vi "I-V_Juliet.vi"() -> ()   [LabVIEW 2013]
uses:
  <vilib>/Utility/file.llb/Read From Spreadsheet File (DBL).vi
panel:
  in  "I-Min":dbl=0.006 format="%#_6e"
  out "dV/dI-I":cluster{dbl[], dbl[]}(graph) caption="XY Graph"
  out "I-V":cluster{dbl[], dbl[]}(graph) caption="XY Graph"
  in  "Measure I-V":bool
  in  "File name":string="C:\\User Data\\Guang\\20201217 Harry 42C\\IV"
  in  "Delta [A]":dbl=1e-05 format="%#_6e"
  in  "Step [A]":dbl=3e-05 format="%#_6e"
  in  "Abort Conductance":bool
  in  "Keithley":refnum<visa-resource-name>="GPIB0::20::INSTR"
  in  "Arm Conductance":bool
  in  "I-Max [A]":dbl=-0.006 format="%#_6e"
  in  "Delay [sec]":dbl=0.002 format="%#_6e"
  in  "Compliance [V]":dbl=10.0 format="%#_6f"
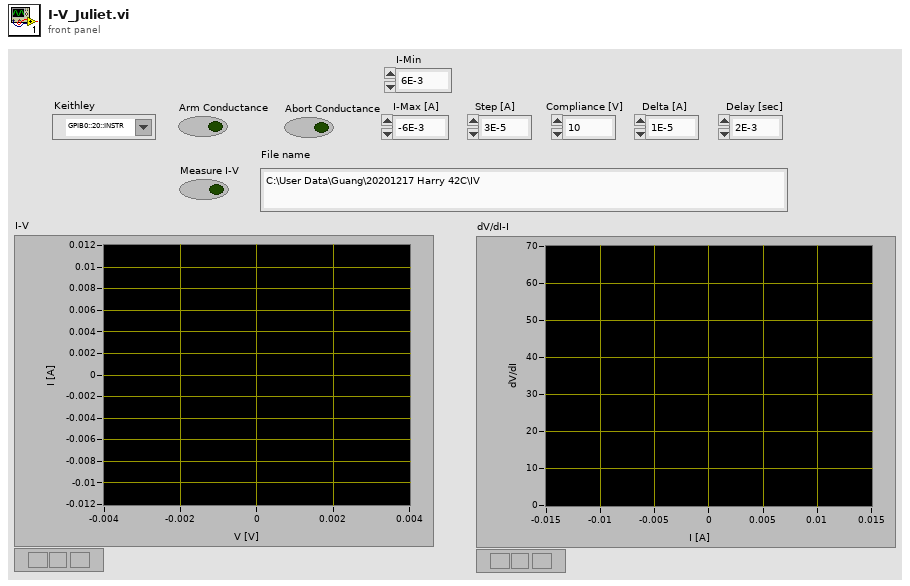
[diagram p1: front panel]
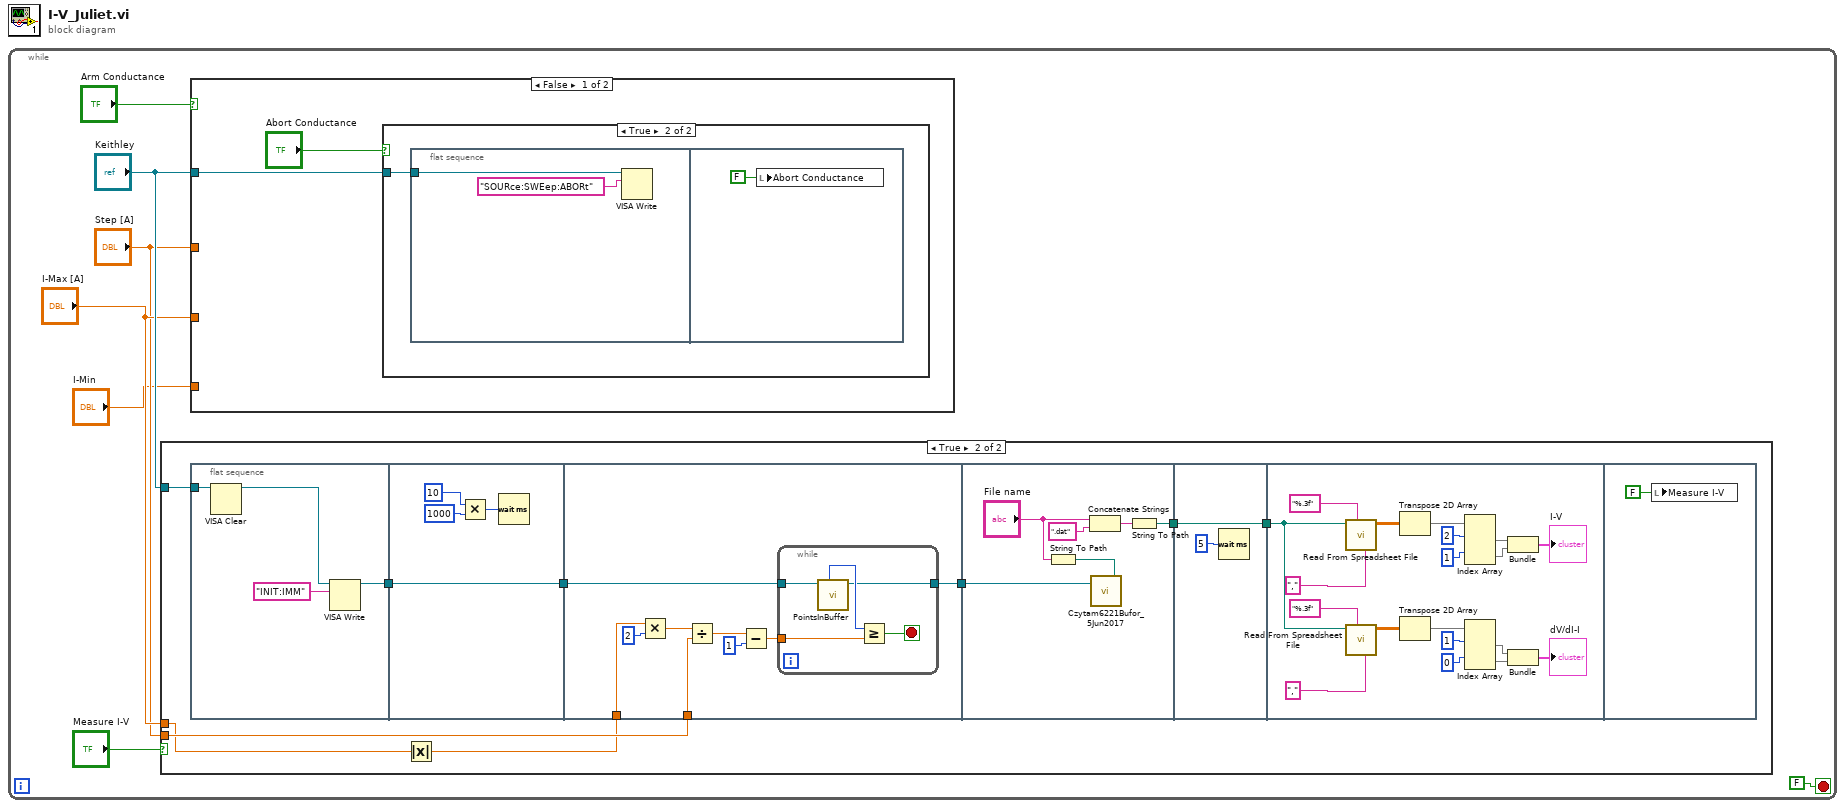
[diagram p0: block diagram]
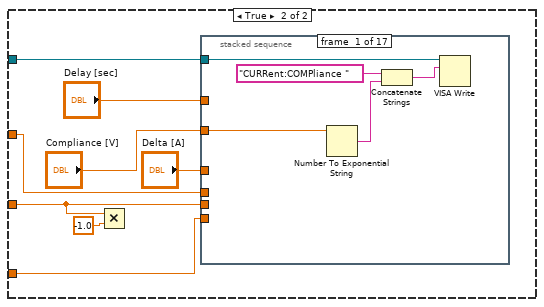
[diagram p4: hidden frame]
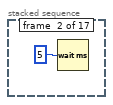
[diagram p5: hidden frame]
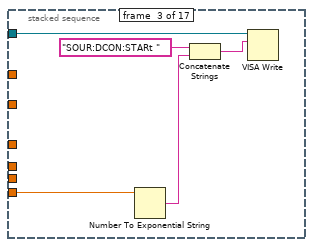
[diagram p6: hidden frame]
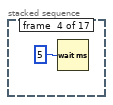
[diagram p7: hidden frame]
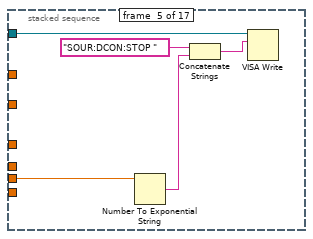
[diagram p8: hidden frame]
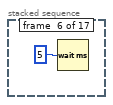
[diagram p9: hidden frame]
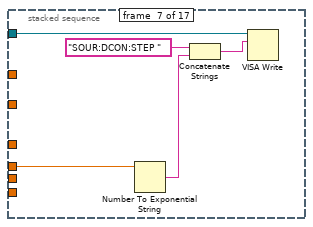
[diagram p10: hidden frame]
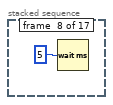
[diagram p11: hidden frame]
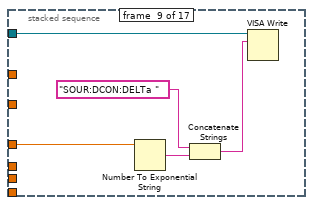
[diagram p12: hidden frame]
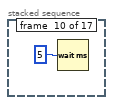
[diagram p13: hidden frame]
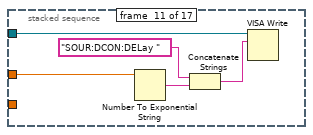
[diagram p14: hidden frame]
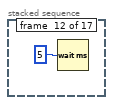
[diagram p15: hidden frame]
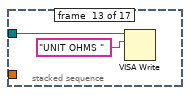
[diagram p16: hidden frame]
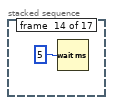
[diagram p17: hidden frame]
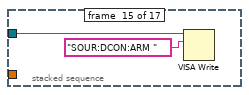
[diagram p18: hidden frame]
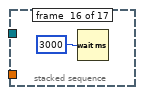
[diagram p19: hidden frame]
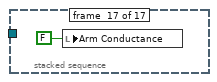
[diagram p20: hidden frame]
diagram:
  n1 = while {
    stop <- FALSE stop-if-true
    n2 = case shown="True" "Measure I-V" {
      tunnel: "Keithley" -> [_ w13]
      tunnel: "I-Max [A]" -> [_ w9]
      tunnel: "Step [A]" -> [_ w12]
      frame False {
      }
      frame True {
        n3 = flat-sequence {
          tunnel: [w18] -> w16
          tunnel: w13 -> [w17]
          tunnel: [w24] -> w15
          tunnel: w16 -> [w24]
          tunnel: w15 -> [w33]
          tunnel: [w32] -> w14
          tunnel: w8 -> [w31]
          tunnel: w12 -> [w28]
          tunnel: w14 -> [w44]
          tunnel: [w41] -> w10
          tunnel: [w45] -> w11
          tunnel: w10 -> [w45]
          tunnel: w11 -> [w47]
          frame #0 {
            n4 = VISA Clear(VISA resource name=w17) -> (VISA resource name out=w20:refnum<visa-resource-name>)  [unwired: 1 in, 1 out]
            n5 = VISA Write(VISA resource name=w20, write buffer="INIT:IMM") -> (VISA resource name out=w18:refnum<visa-resource-name>)  [unwired: 1 in, 2 out]
          }
          frame #1 {
            n6 = Multiply(x=10 ("Waiting time [s]"), y=1000) -> (x*y=w22:i32)
            n7 = Wait (ms)(milliseconds to wait=w22) -> ()  [unwired: 1 out]
          }
          frame #2 {
            n8 = Multiply(x=w31, y=2) -> (x*y=w29:dbl)
            n9 = Divide(x=w29, y=w28) -> (x/y=w27:dbl)
            n10 = Subtract(x=w27, y=1) -> (x-y=w25:dbl)
            n11 = while {
              tunnel: w33 -> [w36]
              tunnel: [w35] -> w32
              tunnel: w25 -> [w34]
              stop <- w37 stop-if-true
              n12 = call "PointsInBuffer.vi"("VISA resource name"=w36) -> (3:w35:refnum<visa-resource-name>, "number"=w38:i32)  [unwired: 9 in]
              n13 = Greater Or Equal?(x=w38, y=w34) -> (x >= y?=w37:bool)
            }
          }
          frame #3 {
            n14 = String To Path(string="File name") -> (path=w43:path)
            n15 = Concatenate Strings("File name", ".dat" ("string")) -> (w42:string)
            n16 = call "Czytam6221Bufor_5Jun2017.vi"("file path (dialog if empty)"=w43, 3:w44) -> ()  [unwired: 1 in, 1 out]
            n17 = String To Path(string=w42) -> (path=w41:path)
          }
          frame #4 {
            n18 = Wait (ms)(milliseconds to wait=u32 5) -> ()  [unwired: 1 out]
          }
          frame #5 {
            n19 = call-poly <vilib>:"Read From Spreadsheet File.vi"("delimiter (\\t)"="," ("delimiter (\\t)"), "format (%.3f)"="%.3f", "file path (dialog if empty)"=w47) -> ("all rows"=w60:dbl[][])  [unwired: 4 in, 4 out]
            n20 = call-poly <vilib>:"Read From Spreadsheet File.vi"("delimiter (\\t)"="," ("delimiter (\\t)"), "format (%.3f)"="%.3f", "file path (dialog if empty)"=w47) -> ("all rows"=w51:dbl[][])  [unwired: 4 in, 4 out]
            n21 = Transpose 2D Array(2D array=w60) -> (transposed array=w59:dbl[][])
            n22 = Transpose 2D Array(2D array=w51) -> (transposed array=w50:dbl[][])
            n23 = Index Array(array=w59, index (row) #1=2 ("index (row)"), index (row) #2=1 ("index (row)")) -> (element #1=w62:dbl[], element #2=w61:dbl[])  [unwired: 2 in]
            n24 = Index Array(array=w50, index (row) #1=1 ("index (row)"), index (row) #2=0 ("index (row)")) -> (element #1=w53:dbl[], element #2=w52:dbl[])  [unwired: 2 in]
            n25 = Bundle(w62, w61) -> (→"I-V":cluster{dbl[], dbl[]})  [unwired: 1 in]
            n26 = Bundle(w53, w52) -> (→"dV/dI-I":cluster{dbl[], dbl[]})  [unwired: 1 in]
          }
          frame #6 {
            n27 = local write "Measure I-V"(FALSE) -> ()
          }
        }
        n28 = Absolute Value(x=w9) -> (abs(x)=w8:dbl)
      }
    }
    n29 = case shown="False" "Arm Conductance" {
      tunnel: "Keithley" -> [w67 w79]
      tunnel: "I-Max [A]" -> [_ w75]
      tunnel: "Step [A]" -> [_ w74]
      tunnel: "I-Min" -> [_ w73]
      frame False {
        n30 = case shown="True" "Abort Conductance" {
          tunnel: w67 -> [_ w69]
          frame False {
          }
          frame True {
            n31 = flat-sequence {
              tunnel: w69 -> [w71]
              frame #0 {
                n32 = VISA Write(VISA resource name=w71, write buffer="SOURce:SWEep:ABORt") -> ()  [unwired: 1 in, 3 out]
              }
              frame #1 {
                n33 = local write "Abort Conductance"(FALSE) -> ()
              }
            }
          }
        }
      }
      frame True {
        n34 = Multiply(x=w75, y=-1.0) -> ()  [unwired: 1 out]
        n35 = stacked-sequence {
          tunnel: w73 -> [_ _ w89 _ _ _ _ _ _ _ _ _ _ _ _ _ _]
          tunnel: w79 -> [w82 _ w87 _ w94 _ w100 _ w106 _ w112 _ w117 _ w120 _ _]
          tunnel: w75 -> [_ _ _ _ w93 _ _ _ _ _ _ _ _ _ _ _ _]
          tunnel: "Delay [sec]" -> [_ _ _ _ _ _ _ _ _ _ w111 _ _ _ _ _ _]
          tunnel: "Compliance [V]" -> [w81 _ _ _ _ _ _ _ _ _ _ _ _ _ _ _ _]
          tunnel: w74 -> [_ _ _ _ _ _ w99 _ _ _ _ _ _ _ _ _ _]
          tunnel: "Delta [A]" -> [_ _ _ _ _ _ _ _ w105 _ _ _ _ _ _ _ _]
          frame #0 {
            n36 = Number To Exponential String(number=w81) -> (E-format string=w84:string)  [unwired: 3 in]
            n37 = Concatenate Strings("CURRent:COMPliance ", w84) -> (w83:string)
            n38 = VISA Write(VISA resource name=w82, write buffer=w83) -> ()  [unwired: 1 in, 3 out]
          }
          frame #1 {
            n39 = Wait (ms)(milliseconds to wait=5) -> ()  [unwired: 1 out]
          }
          frame #2 {
            n40 = Number To Exponential String(number=w89) -> (E-format string=w90:string)  [unwired: 3 in]
            n41 = Concatenate Strings("SOUR:DCON:STARt ", w90) -> (w88:string)
            n42 = VISA Write(VISA resource name=w87, write buffer=w88) -> ()  [unwired: 1 in, 3 out]
          }
          frame #3 {
            n43 = Wait (ms)(milliseconds to wait=5) -> ()  [unwired: 1 out]
          }
          frame #4 {
            n44 = Number To Exponential String(number=w93) -> (E-format string=w96:string)  [unwired: 3 in]
            n45 = Concatenate Strings("SOUR:DCON:STOP ", w96) -> (w95:string)
            n46 = VISA Write(VISA resource name=w94, write buffer=w95) -> ()  [unwired: 1 in, 3 out]
          }
          frame #5 {
            n47 = Wait (ms)(milliseconds to wait=5) -> ()  [unwired: 1 out]
          }
          frame #6 {
            n48 = Number To Exponential String(number=w99) -> (E-format string=w102:string)  [unwired: 3 in]
            n49 = Concatenate Strings("SOUR:DCON:STEP ", w102) -> (w101:string)
            n50 = VISA Write(VISA resource name=w100, write buffer=w101) -> ()  [unwired: 1 in, 3 out]
          }
          frame #7 {
            n51 = Wait (ms)(milliseconds to wait=5) -> ()  [unwired: 1 out]
          }
          frame #8 {
            n52 = Number To Exponential String(number=w105) -> (E-format string=w108:string)  [unwired: 3 in]
            n53 = Concatenate Strings("SOUR:DCON:DELTa ", w108) -> (w107:string)
            n54 = VISA Write(VISA resource name=w106, write buffer=w107) -> ()  [unwired: 1 in, 3 out]
          }
          frame #9 {
            n55 = Wait (ms)(milliseconds to wait=5) -> ()  [unwired: 1 out]
          }
          frame #10 {
            n56 = Number To Exponential String(number=w111) -> (E-format string=w114:string)  [unwired: 3 in]
            n57 = Concatenate Strings("SOUR:DCON:DELay ", w114) -> (w113:string)
            n58 = VISA Write(VISA resource name=w112, write buffer=w113) -> ()  [unwired: 1 in, 3 out]
          }
          frame #11 {
            n59 = Wait (ms)(milliseconds to wait=5) -> ()  [unwired: 1 out]
          }
          frame #12 {
            n60 = VISA Write(VISA resource name=w117, write buffer="UNIT OHMS ") -> ()  [unwired: 1 in, 3 out]
          }
          frame #13 {
            n61 = Wait (ms)(milliseconds to wait=5) -> ()  [unwired: 1 out]
          }
          frame #14 {
            n62 = VISA Write(VISA resource name=w120, write buffer="SOUR:DCON:ARM ") -> ()  [unwired: 1 in, 3 out]
          }
          frame #15 {
            n63 = Wait (ms)(milliseconds to wait=3000) -> ()  [unwired: 1 out]
          }
          frame #16 {
            n64 = local write "Arm Conductance"(FALSE) -> ()
          }
        }
      }
    }
  }
